vi "LVClass_Image ctor.vi"(0 "Image in":refnum<class "Image.lvclass">, 7 "Data alignment":T1=enum."16", 9 "Size":T2, 11 "error in (no error)":errorcluster) -> (4 "Image out":refnum<class "Image.lvclass">, 15 "error out":errorcluster)   [LabVIEW 2020, in "Image.lvclass"]
doc: "Single channel Image constructor from dimensions and bit depth.\n\n--------------------------------------------------------------------------------\n\n<B>ImageIn </B> : Constant Pointer to Image object.\n<B>ImageOut </B> : Constant Pointer to Image object.\n<B>size </B> : 2D image size.\n<B>bit_depth </B> : Image bits depth.\n<B>ErrorIn </B> : Error\n<B>ErrorOut </B> : Error\n\n--------------------------------------------------------------------------------"
uses:
  Image.lvclass
  Point2D.ctl
  Data alignment enum.ctl
  Handle creation.ctl
  Image.lvclass/Image.ctl
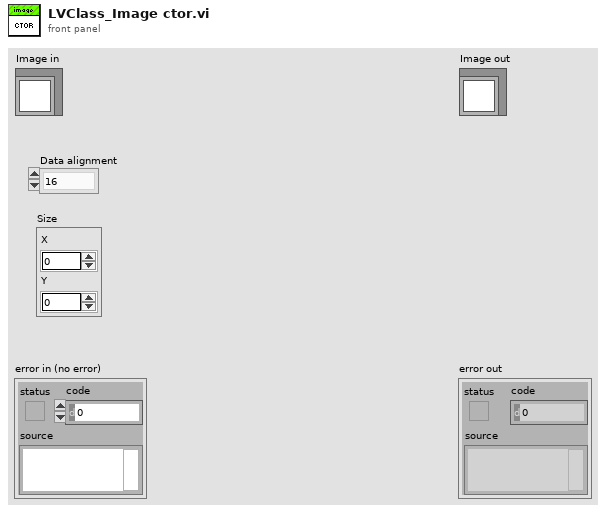
[diagram p1: front panel]
types:
  T1 = typedef "Data alignment enum.ctl" = enum16{"8", "16", "32"}
  T2 = typedef "Point2D.ctl" = cluster{"X":u32, "Y":u32}
  T3 = typedef "Handle creation.ctl" = enum16{"By ctor", "By write function"}
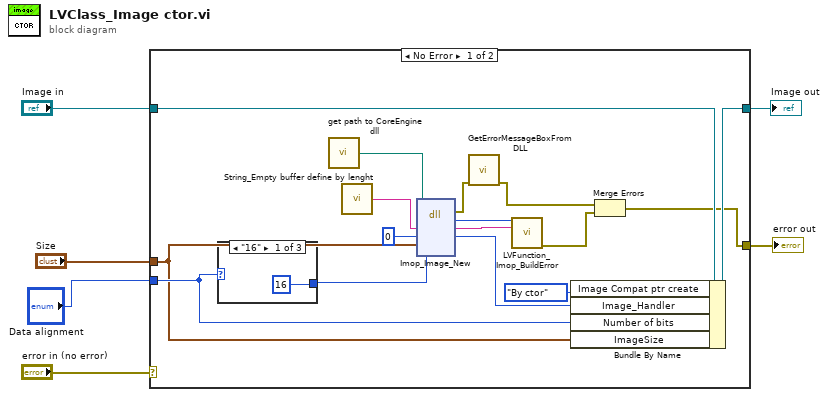
[diagram p0: block diagram]
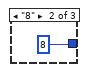
[diagram p2: hidden frame]
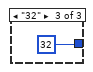
[diagram p3: hidden frame]
diagram:
  n1 = case shown="No Error" "error in (no error)" {
    selector: "error in (no error)" -> [_ w27]
    tunnel: [w7 w27] -> w5
    tunnel: [w18 w26] -> w3
    tunnel: "Image in" -> [w19 w26]
    tunnel: "Size" -> [w11 _]
    tunnel: "Data alignment" -> [w12 _]
    frame No Error {
      n2 = case shown="\"16\"" w12 {
        tunnel: [u16 16 ("Image compat") u16 8 ("Image compat") u16 32 ("Image compat")] -> w13
        frame "16" {
        }
        frame "8" {
        }
        frame "32" {
        }
      }
      n3 = call "get path to CoreEngine dll.vi"() -> ("path to c_interface_vc100.dll"=w15:path)  [unwired: 12 in, 3 out]
      n4 = call "String_Empty buffer define by lenght.vi"() -> ("Empty buffer"=w20:string)  [unwired: 1 in]
      n5 = dll-call lib="D:/soft/HASO_v3/SVN_trunk/ImOpCoreEngine4_LV2011/DLLs/c_interface_vc100.dll" fn="Imop_Image_New"(path in=w15, "message"=w20, "Image compat"=0, "Size"=w11, "Nb_Bits"=w13) -> (error out=w14:errorcluster, "return type"=w21:i32, "message"=w22:string, "Image compat"=w10:i32)  [unwired: 4 in, 1 out]
      n6 = call "GetErrorMessageBoxFromDLL.vi"("error IN"=w14) -> ("error OUT"=w9:errorcluster)  [unwired: 10 in]
      n7 = call "LVFunction_Imop_BuildError.vi"("code"=w21, "String to Prepend to source (\"\")"=w22) -> ("error out"=w8:errorcluster)  [unwired: 13 in]
      n8 = Bundle By Name(cluster=w19, "Image Compat ptr create"=Handle_creation."By ctor", "Image_Handler"=w10, "Number of bits"=w12, "ImageSize"=w11) -> (w18:refnum<class "Image.lvclass">)
      n9 = Merge Errors(w9, w8) -> (w7:errorcluster)
    }
    frame Error {
    }
  }
  "error out" <- w5
  "Image out" <- w3
